vi "String to I64.vi"(1 "String":string) -> (0 "I64":i64)   [LabVIEW 2011]
doc: "Convert string to number. Small VI to be block-diagram friendly.\n\nVersion 1.0 - 09/13/2013\n\nPhaeron, Inc.\nwww.phaeron.com\ninfo@phaeron.com"
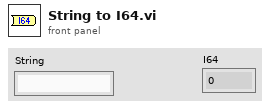
[diagram p1: front panel]
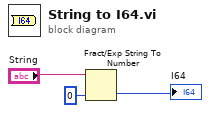
[diagram p0: block diagram]
diagram:
  n1 = Fract/Exp String To Number(string="String", default (0 dbl)=i64 0 ("default (0 DBL)")) -> (number=→"I64":i64)  [unwired: 2 in, 1 out]
